vi "TIFF ULS to File mk2.vi"(5 "Image Size":u32, 7 "Layer Count":i32, 8 "error in (no error)":errorcluster, 9 "Basic IFD":refnum<class "IFD.lvclass">, 10 "refnum in":refnum<file>, 11 "TIFF ULS in":refnum<class "TIFF ULS.lvclass">) -> (0 "error out":errorcluster, 1 "Reference Offset":u32, 2 "refnum out":refnum<file>)   [LabVIEW 2016, in "TIFF ULS.lvclass"]
uses:
  TIFF ULS.lvclass
  IFD/IFD.lvclass
  TIFF ULS.lvclass/TIFF ULS.ctl
  IFD/IFD.lvclass/IFD.ctl
  Tag/IFD_Tag.lvclass/IFD_Tag.ctl
  Tag/Tag Size.vi
  Tag/Tag Write to File.vi
  IFD/Write All Pending Data.vi
  Tag/IFD_Tag.lvclass
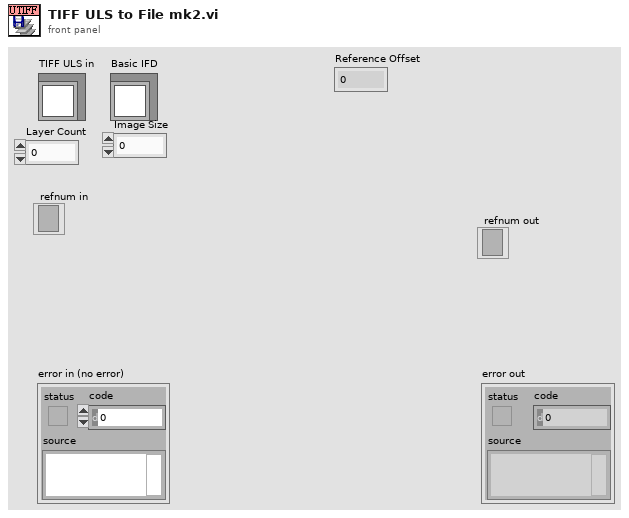
[diagram p1: front panel]
types:
  T1 = enum16{"big-endian, network order", "native, host order", "little-endian"}
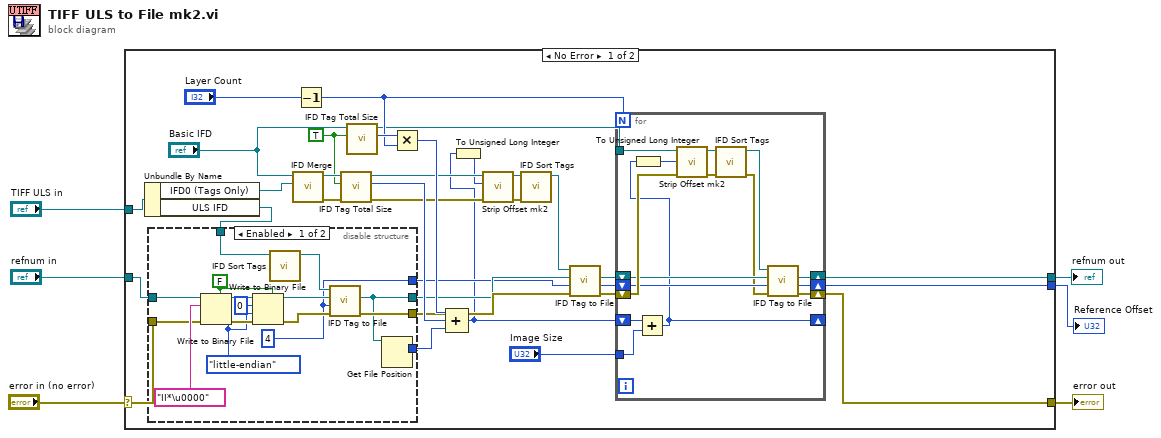
[diagram p0: block diagram]
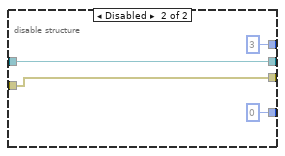
[diagram p2: hidden frame]
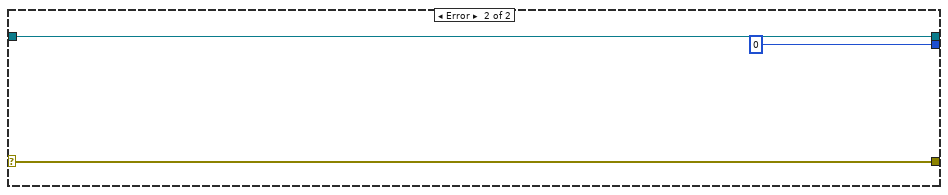
[diagram p3: hidden frame]
diagram:
  n1 = case shown="No Error" "error in (no error)" {
    selector: "error in (no error)" -> [w36 w77]
    tunnel: [w35 w77] -> w5
    tunnel: "TIFF ULS in" -> [w38 _]
    tunnel: "refnum in" -> [w37 w76]
    tunnel: [w11 w76] -> w2
    tunnel: [w13 u32 0 ("Reference Offset")] -> w1
    frame No Error {
      w12 = TRUE ("Add Strip")
      n2 = Unbundle By Name(w38) -> ("IFD0 (Tags Only)"=w39:refnum<class "IFD.lvclass">, "ULS IFD"=w7:refnum<class "IFD.lvclass">)
      n3 = disable-structure shown="Enabled" {
        disable-tunnel: w37 -> [w48 w59]
        disable-tunnel: w36 -> [w47 w58]
        disable-tunnel: [w45 i64 0 ("offset (in bytes)")] -> w31
        disable-tunnel: [w44 w58] -> w23
        disable-tunnel: [w43 w59] -> w21
        disable-tunnel: [w42 u32 3 ("Last Reference Offset")] -> w18
        disable-tunnel: w7 -> [w40 _]
        frame Enabled {
          w41 = T1."little-endian" ("byte order (0:big-endian, network order)")
          w42 = u32 4 ("Last Reference Offset")
          w46 = FALSE ("prepend array or string size? (T)")
          n4 = Write to Binary File(file (use dialog)=w48, data="II*\u0000", error in=w47, 5:w46, 9:w41) -> (refnum out=w54:refnum<file>, error out=w52:errorcluster)  [unwired: 2 out]
          n5 = Write to Binary File(file (use dialog)=w54, data=u32 0, error in=w52, 5:w46, 9:w41) -> (refnum out=w50:refnum<file>, error out=w51:errorcluster)  [unwired: 2 out]
          n6 = call "IFD Sort Tags.vi"("IFD in"=w40) -> ("IFD out"=w49:refnum<class "IFD.lvclass">)  [unwired: 9 in, 1 out]
          n7 = call "IFD Tag to File.vi"("error in (no error)"=w51, "Last Reference Offset"=w42, "refnum in"=w50, "IFD in"=w49) -> ("error out"=w44:errorcluster, "refnum out"=w43:refnum<file>)  [unwired: 4 in, 2 out]
          n8 = Get File Position(7:w43) -> (2:w45:i64)  [unwired: 1 in, 2 out]
        }
        frame Disabled {
        }
      }
      n9 = call "IFD Merge.vi"("subIFD"=w39, "main IFD"="Basic IFD") -> ("error out"=w16:errorcluster, "IFD out"=w33:refnum<class "IFD.lvclass">)  [unwired: 8 in]
      n10 = Decrement(x="Layer Count") -> (x-1=w28:i32)
      n11 = call "IFD Tag Total Size.vi"("error in (no error)"=w16, "Add Strip"=w12, "IFD in"=w33) -> ("error out"=w15:errorcluster, "Size(byte)"=w30:u32, "IFD out"=w25:refnum<class "IFD.lvclass">)  [unwired: 6 in]
      n12 = call "IFD Tag Total Size.vi"("Add Strip"=w12, "IFD in"="Basic IFD") -> ("Size(byte)"=w29:u32, "IFD out"=w26:refnum<class "IFD.lvclass">)  [unwired: 7 in, 1 out]
      n13 = Multiply(x=w29, y=w28) -> (x*y=w27:u32)
      n14 = Compound Arithmetic op=ADD(w27, w30, w31) -> (w9:i64)
      n15 = To Unsigned Long Integer(number=w9) -> (unsigned 32bit integer=w8:u32)
      n16 = call "Strip Offset mk2.vi"("error in (no error)"=w15, "Offset"=w8, "IFD in"=w25) -> ("error out"=w14:errorcluster, "IFD out"=w24:refnum<class "IFD.lvclass">)  [unwired: 7 in]
      n17 = call "IFD Sort Tags.vi"("error in (no error)"=w14, "IFD in"=w24) -> ("IFD out"=w19:refnum<class "IFD.lvclass">)  [unwired: 8 in, 1 out]
      n18 = call "IFD Tag to File.vi"("error in (no error)"=w23, "Last Reference Offset"=w18, "refnum in"=w21, "IFD in"=w19) -> ("error out"=w22:errorcluster, "Reference Offset"=w10:u32, "refnum out"=w20:refnum<file>)  [unwired: 4 in, 1 out]
      n19 = for {
        N: w28 -> [_]
        shift-right: [w64] -> w35
        shift-left: w22 -> [w71]
        shift-right: [w62] -> w11
        shift-left: w20 -> [w68]
        shift-right: [w63] -> w13
        shift-left: w10 -> [w66]
        shift-right: [w61] -> _
        shift-left: w9 -> [w74]
        tunnel: w26 -> [w72]
        tunnel: "Image Size" -> [w73]
        n20 = Add(x=w74, y=w73) -> (x+y=w61:i64)
        n21 = To Unsigned Long Integer(number=w61) -> (unsigned 32bit integer=w60:u32)
        n22 = call "Strip Offset mk2.vi"("error in (no error)"=w71, "Offset"=w60, "IFD in"=w72) -> ("error out"=w69:errorcluster, "IFD out"=w70:refnum<class "IFD.lvclass">)  [unwired: 7 in]
        n23 = call "IFD Sort Tags.vi"("error in (no error)"=w69, "IFD in"=w70) -> ("error out"=w65:errorcluster, "IFD out"=w67:refnum<class "IFD.lvclass">)  [unwired: 8 in]
        n24 = call "IFD Tag to File.vi"("error in (no error)"=w65, "Last Reference Offset"=w66, "refnum in"=w68, "IFD in"=w67) -> ("error out"=w64:errorcluster, "Reference Offset"=w63:u32, "refnum out"=w62:refnum<file>)  [unwired: 4 in, 1 out]
      }
    }
    frame Error {
    }
  }
  "error out" <- w5
  "refnum out" <- w2
  "Reference Offset" <- w1
